vi "lv_opencv_demo.vi"() -> ()   [LabVIEW 2021]
uses:
  <vilib>/vision/NI_Vision_Development_Module.lvlib
panel:
  in  "dll_Path":path
  in  "img_Path":path
  out "输出图像":T1(plugin-control)
  out "Original":T1(plugin-control)
  # "[class_id, score, x1, y1, x2, y2]"
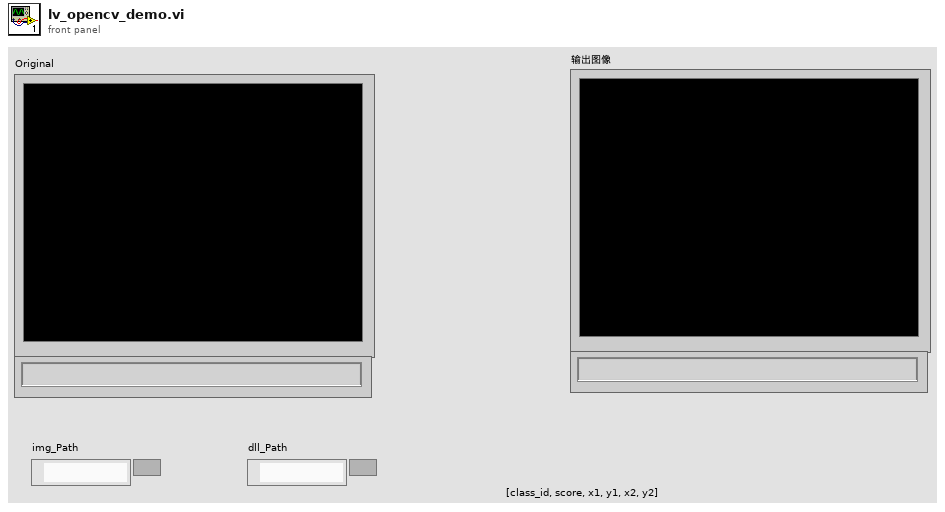
[diagram p1: front panel]
types:
  T1 = typedef "IMAQ Image.ctl" = refnum<image>
  T2 = typedef "Image Type" = u32
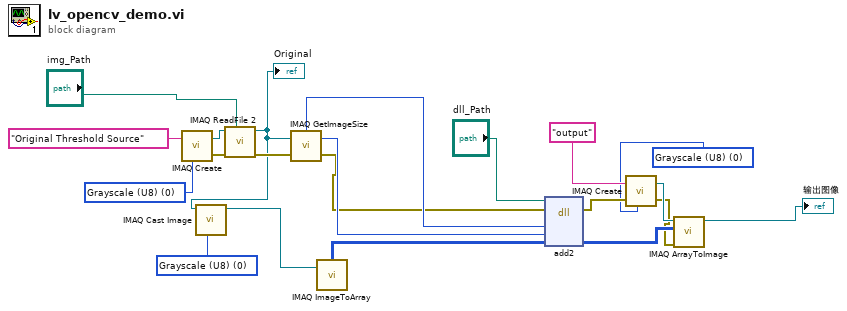
[diagram p0: block diagram]
diagram:
  w4 = T2 0 items=["Grayscale (U8)", "Grayscale (I16)", "Grayscale (SGL)", "Complex (CSG)", "RGB (U32)", "HSL (U32)", "RGB (U64)", "Grayscale (U16)"] ("Image Type")
  w10 = T2 0 items=["Grayscale (U8)", "Grayscale (I16)", "Grayscale (SGL)", "Complex (CSG)", "RGB (U32)", "HSL (U32)", "RGB (U64)", "Grayscale (U16)"] ("Image Type")
  w18 = T2 0 items=["Grayscale (U8)", "Grayscale (I16)", "Grayscale (SGL)", "Complex (CSG)", "RGB (U32)", "HSL (U32)", "RGB (U64)", "Grayscale (U16)"] ("Image Type")
  n1 = call "IMAQ Create"("Image Name"="Original Threshold Source", "Image Type"=w18) -> ("New Image"=w20:T1, "error out"=w19:errorcluster)  [unwired: 3 in]
  n2 = call "IMAQ ReadFile 2"("File Path"="img_Path", "error in (no error)"=w19, "Image"=w20) -> ("error out"=w15:errorcluster, "Image Out"=w3:T1)  [unwired: 4 in, 3 out]
  "Original" <- w3
  n3 = call "IMAQ Cast Image"("Image Type"=w4, "Image Src"=w3) -> ("Image Dst Out"=w2:T1)  [unwired: 8 in, 1 out]
  n4 = call "IMAQ GetImageSize"("Image"=w3, "error in (no error)"=w15) -> ("Y Resolution"=w16:i32, "X Resolution"=w17:i32, "error out"=w14:errorcluster)  [unwired: 2 in]
  n5 = call "IMAQ ImageToArray"("Image"=w2) -> ("Image Pixels (U8)"=w13:u8[][])  [unwired: 3 in, 4 out]
  n6 = dll-call lib="E:/projects/cppProjects/ppyolov2_openvino_samples/lv2cv.dll" fn="add2"(path in="dll_Path", error in=w14, "rows"=w17, "cols"=w16, "data"=w13) -> (error out=w12:errorcluster, "data"=w9:u8[][])  [unwired: 4 in, 1 out]
  n7 = call "IMAQ Create"("Image Name"="output", "Image Type"=w10, "error in (no error)"=w12) -> ("New Image"=w8:T1, "error out"=w1:errorcluster)  [unwired: 2 in]
  n8 = call "IMAQ ArrayToImage"("error in (no error)"=w1, "Image Pixels (U8)"=w9, "Image"=w8) -> ("Image Out"=→"输出图像":T1)  [unwired: 7 in, 1 out]
